vi "Count Down.vi"() -> ()   [LabVIEW 2012]
panel:
  out "count":i32
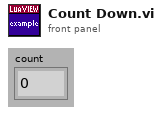
[diagram p1: front panel]
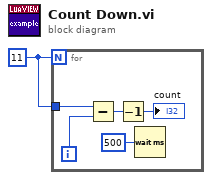
[diagram p0: block diagram]
diagram:
  w1 = 11
  n1 = for {
    N: w1 -> [_]
    tunnel: w1 -> [w5]
    i -> [w4]
    n2 = Subtract(x=w5, y=w4) -> (x-y=w3:i32)
    n3 = Decrement(x=w3) -> (x-1=→"count":i32)
    n4 = Wait (ms)(milliseconds to wait=u32 500) -> ()  [unwired: 1 out]
  }
